vi "add.issues.vi"(0 "issues in":map{i32, T1}(c390), 1 "Array":path[](array[path]), 5 "char map in":T2, 7 "concept map in":T2, 9 "story map in":T2, 11 "error in (no error)":errorcluster, 12 "team map in":T2) -> (4 "issues out":map{i32, T1}(c390), 6 "char map out":T2, 8 "concept map out":T2, 10 "story map out":T2, 14 "team map out":T2, 15 "error out":errorcluster)   [LabVIEW 2024, in "manager_daemon.lvclass"]
uses:
  manager_daemon.lvclass
  manager_daemon.lvclass/manager_daemon.ctl
  type_defs/IssueData--clustrer.ctl
  type_defs/SubData--cluster.ctl
  type_defs/sub-map--map.ctl
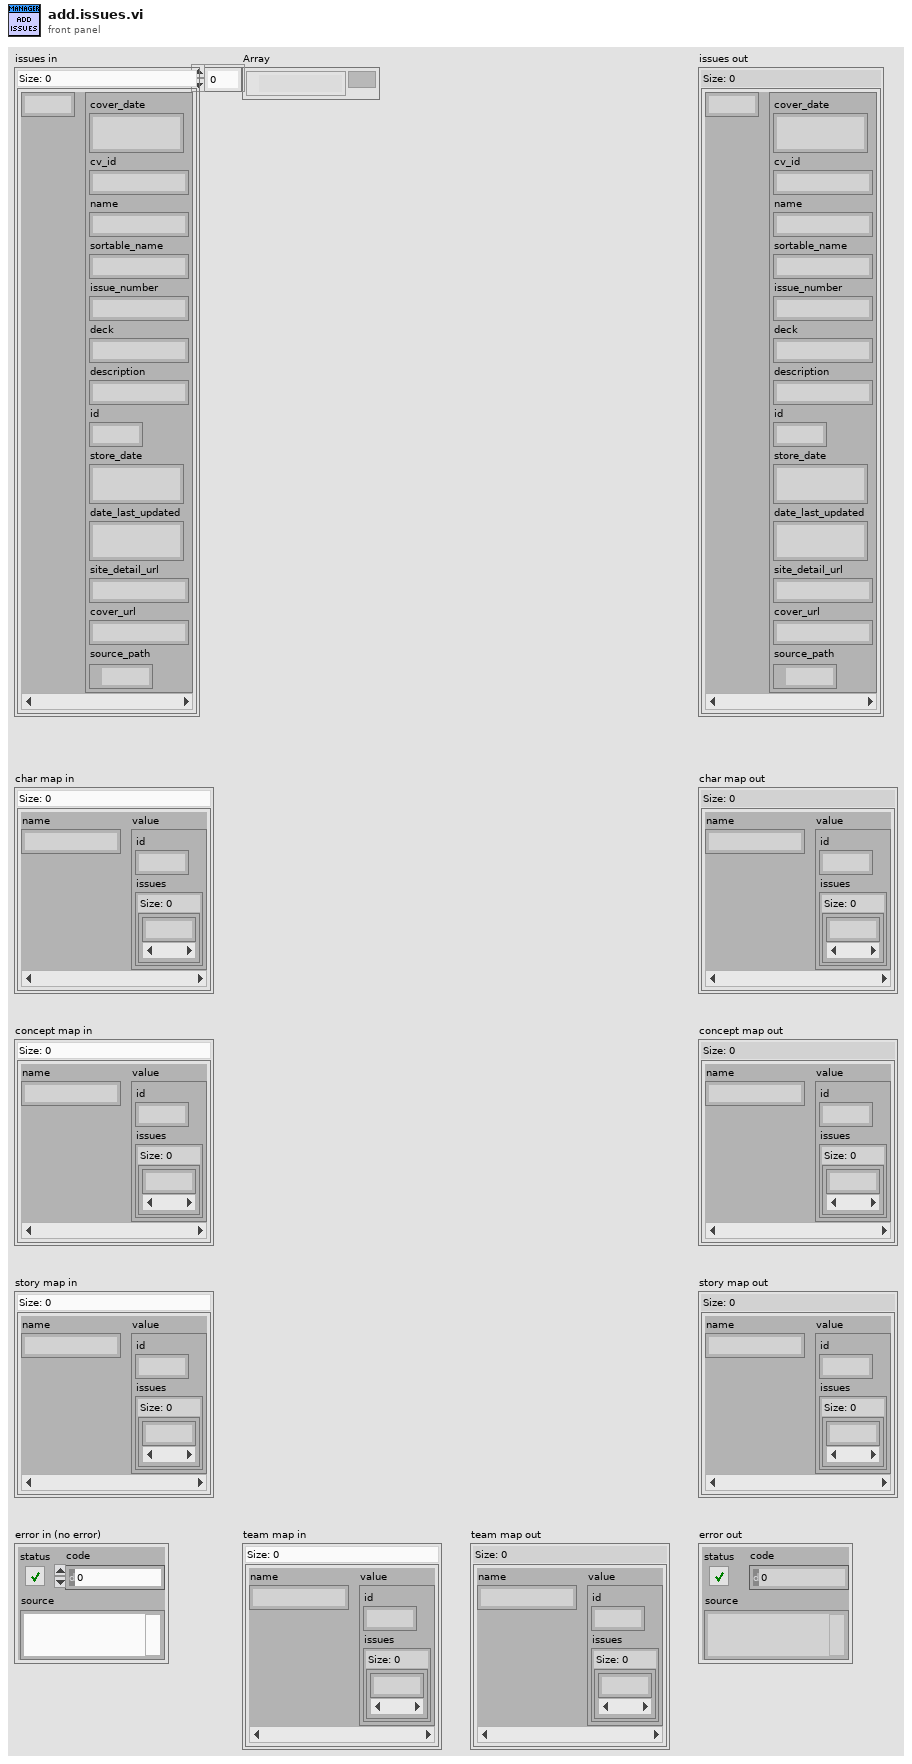
[diagram p1: front panel]
types:
  T1 = typedef "manager_daemon.lvclass/IssueData--clustrer.ctl" = cluster{"cover_date":timestamp, "cv_id":string, "name":string, "sortable_name":string, "issue_number":string, "deck":string, "description":string, "id":i32, "store_date":timestamp, "date_last_updated":timestamp, "site_detail_url":string, "cover_url":string, "source_path":path}
  T2 = typedef "manager_daemon.lvclass/sub-map--map.ctl" = map{string, T3}
  T3 = typedef "manager_daemon.lvclass/SubData--cluster.ctl" = cluster{"id":i32, "issues":set{i32}}
  T4 = typedef "local_issue.ctl" = cluster{"cover_date":timestamp, "id":i32, "cv_id":string, "name":string, "sortable_name":string, "issue_number":string, "deck":string, "description":string, "volume":T5, "store_date":timestamp, "date_last_updated":timestamp, "site_detail_url":string, "cover_url":string, "associated_images":T6[], "characters":T5[], "concepts":T5[], "creators":T7[], "storyArcs":T5[], "teams":T5[]}
  T5 = typedef "comicvine_issue.generic_credit.ctl" = cluster{"id":i32, "name":string}
  T6 = typedef "comicvine_issue.associated_image.ctl" = cluster{"original_url":string, "id":i32}
  T7 = typedef "comicvine_issue.person_credit.ctl" = cluster{"id":i32, "name":string, "role":string}
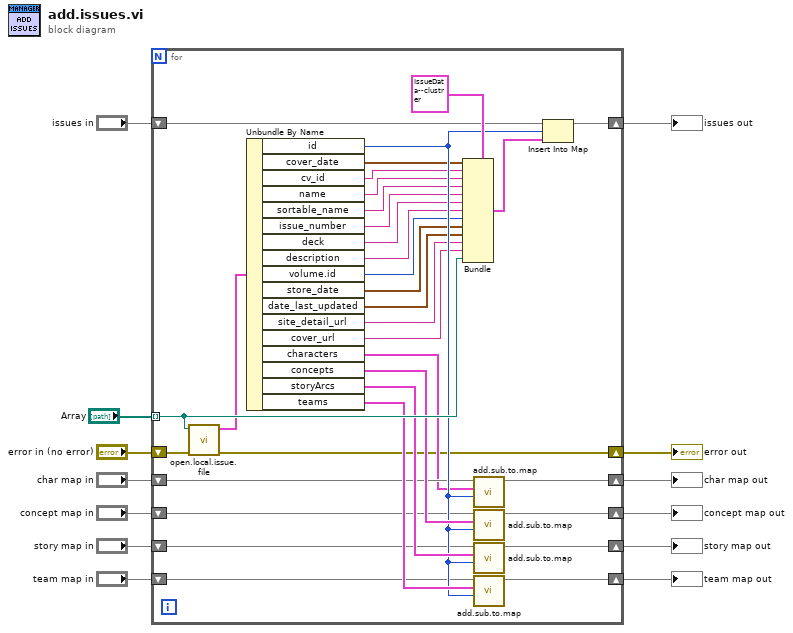
[diagram p0: block diagram]
diagram:
  n1 = for {
    tunnel: "Array" -> [w45] mode=indexing
    shift-right: [w31] -> w4
    shift-left: "error in (no error)" -> [w14]
    shift-right: [w30] -> w3
    shift-left: "issues in" -> [w28]
    shift-right: [w33] -> w5
    shift-left: "char map in" -> [w34]
    shift-right: [w38] -> w10
    shift-left: "concept map in" -> [w35]
    shift-right: [w39] -> w11
    shift-left: "story map in" -> [w36]
    shift-right: [w40] -> w12
    shift-left: "team map in" -> [w37]
    n2 = call "open.local.issue.file.vi"("error in (no error)"=w14, "volume json"=w45) -> ("error out"=w31:errorcluster, "issue"=w15:T4)  [unwired: 8 in]
    n3 = Unbundle By Name(w15) -> ("id"=w41:i32, "cover_date"=w16:timestamp, "cv_id"=w17:string, "name"=w18:string, "sortable_name"=w19:string, "issue_number"=w20:string, "deck"=w21:string, "description"=w22:string, "volume.id"=w23:i32, "store_date"=w24:timestamp, "date_last_updated"=w25:timestamp, "site_detail_url"=w26:string, "cover_url"=w27:string, "characters"=w32:T5[], "concepts"=w42:T5[], "storyArcs"=w43:T5[], "teams"=w44:T5[])
    n4 = Bundle(cluster=T1 {"cover_date"=timestamp(0 s since 1904-01-01), "cv_id"="", "name"="", "sortable_name"="", "issue_number"="", "deck"="", "description"="", "id"=0, "store_date"=timestamp(0 s since 1904-01-01), "date_last_updated"=timestamp(0 s since 1904-01-01), "site_detail_url"="", "cover_url"="", "source_path"=path ""} ("issue data"), "cover_date"=w16, "cv_id"=w17, "name"=w18, "sortable_name"=w19, "issue_number"=w20, "deck"=w21, "description"=w22, "id"=w23, "store_date"=w24, "date_last_updated"=w25, "site_detail_url"=w26, "cover_url"=w27, "source_path"=w45) -> (w29:T1)
    n5 = call "add.sub.to.map.vi"("id"=w41, "data"=w32, "map out"=w34) -> ("map out"=w33:T2)  [unwired: 8 in]
    n6 = call "add.sub.to.map.vi"("id"=w41, "data"=w42, "map out"=w35) -> ("map out"=w38:T2)  [unwired: 8 in]
    n7 = call "add.sub.to.map.vi"("id"=w41, "data"=w43, "map out"=w36) -> ("map out"=w39:T2)  [unwired: 8 in]
    n8 = call "add.sub.to.map.vi"("id"=w41, "data"=w44, "map out"=w37) -> ("map out"=w40:T2)  [unwired: 8 in]
    n9 = Insert Into Map(map in=w28, key=w41, value=w29) -> (map out=w30:map{i32, T1})  [unwired: 2 out]
  }
  "team map out" <- w12
  "story map out" <- w11
  "concept map out" <- w10
  "char map out" <- w5
  "error out" <- w4
  "issues out" <- w3
